vi "TimeOut+ForceTrigger.vi"(8 "error in (no error)":errorcluster, 9 "lines per plane mod":i32, 10 "Timeout (10000 ms)":u32=10000, 11 "VISA resource name":refnum<visa-resource-name>) -> (0 "error out":errorcluster, 1 "Missing Lines":i32, 2 "Complete":bool, 3 "VISA resource name out":refnum<visa-resource-name>)   [LabVIEW 2022 SP3]
uses:
  <instrlib>/LeCroy Wave Series/LeCroy Wave Series.lvlib
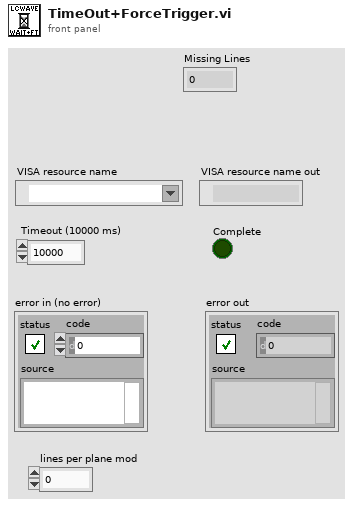
[diagram p1: front panel]
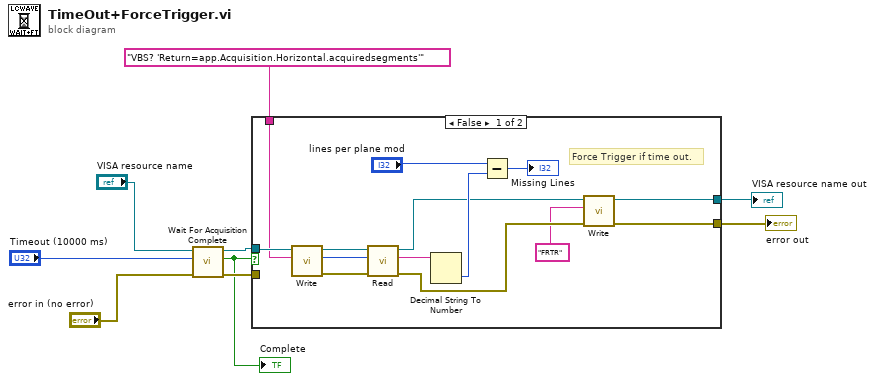
[diagram p0: block diagram]
diagram:
  n1 = call <instrlib>:"Wait For Acquisition Complete.vi"("error in (no error)"="error in (no error)", "Timeout (10000 ms)"="Timeout (10000 ms)", "VISA resource name"="VISA resource name") -> ("error out"=w6:errorcluster, "Complete"=w2:bool, "VISA resource name out"=w4:refnum<visa-resource-name>)  [unwired: 6 in]
  "Complete" <- w2
  n2 = case shown="False" w2 {
    tunnel: w6 -> [_ w24]
    tunnel: [w13 w25] -> w5
    tunnel: w4 -> [w21 w25]
    tunnel: [w14 w24] -> w3
    tunnel: "VBS? 'Return=app.Acquisition.Horizontal.acquiredsegments'" ("Write Buffer") -> [w18 _]
    frame False {
      # "Force Trigger if time out."
      n3 = call <instrlib>:"Write.vi"("Write Buffer"=w18, "VISA resource name"=w21) -> ("error out"=w22:errorcluster, "Return Count"=w20:u32, "VISA resource name out"=w23:refnum<visa-resource-name>)  [unwired: 7 in]
      n4 = call <instrlib>:"Read.vi"("error in (no error)"=w22, "Byte Count"=w20, "VISA resource name"=w23) -> ("error out"=w15:errorcluster, "Read Buffer"=w19:string, "VISA resource name out"=w12:refnum<visa-resource-name>)  [unwired: 5 in, 1 out]
      n5 = Decimal String To Number(string=w19) -> (number=w16:i32)  [unwired: 2 in, 1 out]
      n6 = Subtract(x="lines per plane mod", y=w16) -> (x-y=→"Missing Lines":i32)
      n7 = call <instrlib>:"Write.vi"("error in (no error)"=w15, "Write Buffer"="FRTR", "VISA resource name"=w12) -> ("error out"=w14:errorcluster, "VISA resource name out"=w13:refnum<visa-resource-name>)  [unwired: 6 in, 1 out]
    }
    frame True {
    }
  }
  "VISA resource name out" <- w5
  "error out" <- w3
